vi "Enable Streaming.vi"(8 "error in (no error)":errorcluster, 11 "Node Ptr":T1 format="%.0x") -> (0 "error out":errorcluster)   [LabVIEW 2024, in "Nominal Client System Explorer.lvlib"]
uses:
  Nominal Client System Explorer.lvlib
  <vilib>/NI VeriStand/Custom Device API/Custom Device Item Ref.ctl
  <vilib>/NI VeriStand/Custom Device API/Custom Device API.lvlib
panel:
  in  "Specific Header":cluster{"Section Name":string}={"Section Name"="Specific Page Settings"}
  in  "General Header":cluster{"Section Name":string}={"Section Name"="General Page Settings"}
  in  "Description":string
  in  "Name":string
  # "Overview\nThe system provides a data channel that controls whether data is streamed to a file. This channel accepts float values but functions as a Boolean control.\n\nHow It Works\nChannel Value = 0: Streaming is disabled (False)\nChannel Value != 0: Streaming is enabled (True)\n\nUsage Methods\nManual Control\nPlace a Button on the User Interface screen and link it to:\n`Nominal IO VeriStand Client\\Enable Streaming`\nThis provides direct manual control over the streaming functionality.\n\nDynamic Control\nYou can also incorporate the channel in calculations to automatically control streaming based on other conditions or system states."
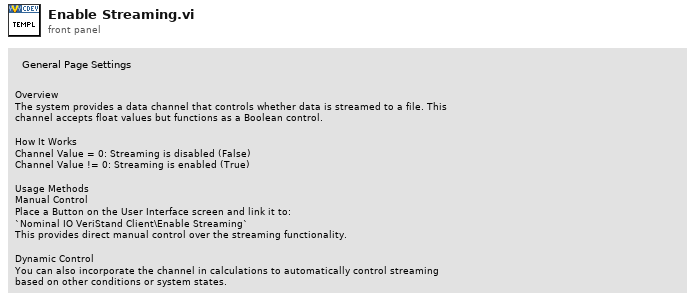
[diagram p1: front panel]
types:
  T1 = typedef "Custom Device API.lvlib/Custom Device Item Ref.ctl" = u64
  T2 = typedef "Custom Device API.lvlib/Custom Device Item Info.ctl" = cluster{"Name":string, "Is Channel":bool, "GUID":string, "Is Waveform":bool}
  T3 = typedef "Custom Device API.lvlib/Custom Device Commands.ctl" = enum16{"Default", "Item renamed", "Shutdown", "Dynamic button pressed"}
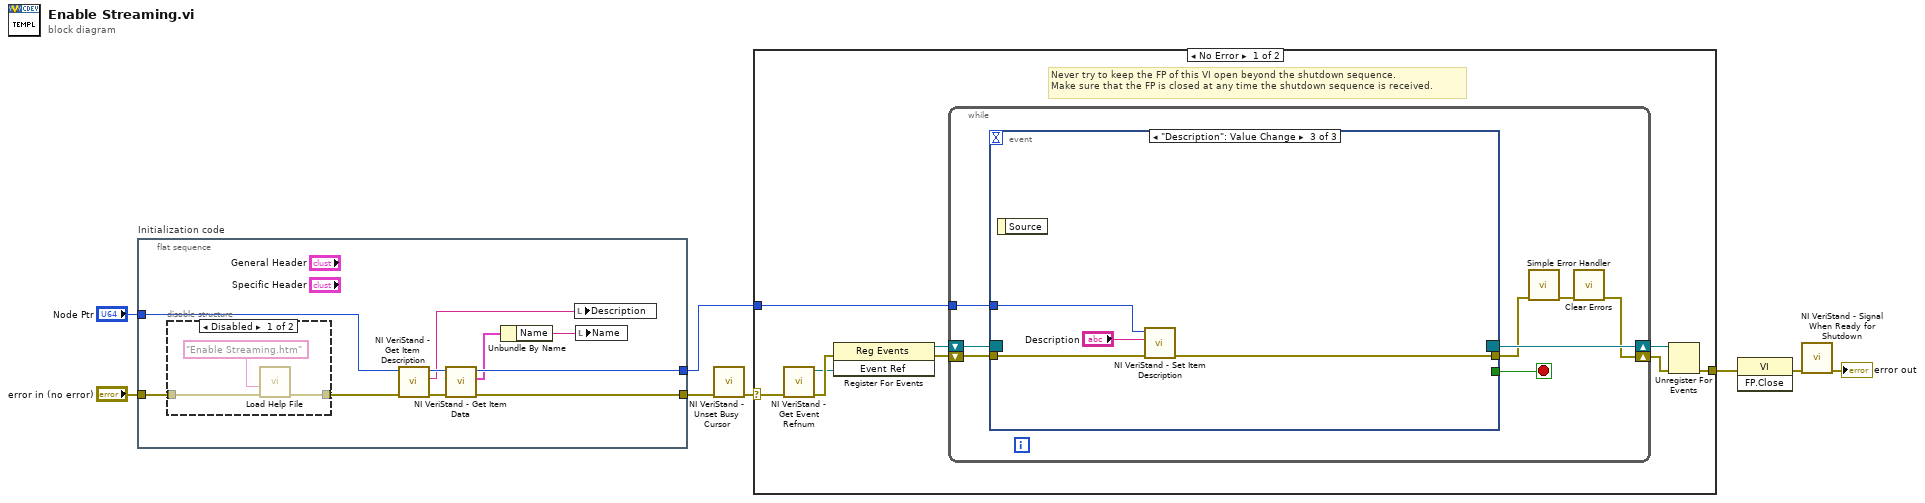
[diagram p0: block diagram]
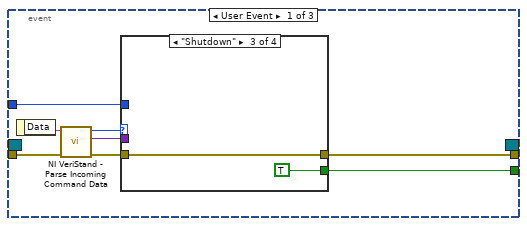
[diagram p2: hidden frame]
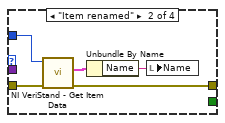
[diagram p4: hidden frame]
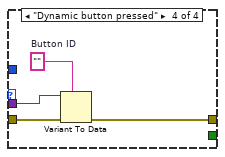
[diagram p5: hidden frame]
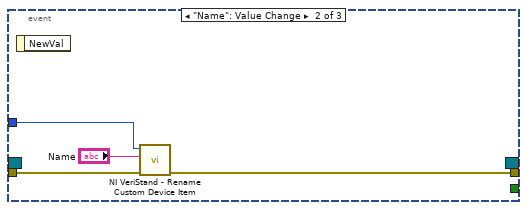
[diagram p6: hidden frame]
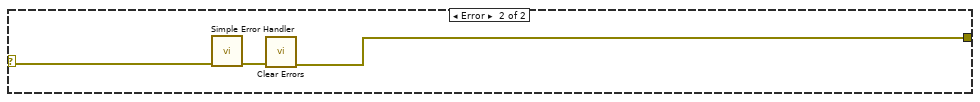
[diagram p7: hidden frame]
diagram:
  n1 = flat-sequence "Initialization code" {
    tunnel: "error in (no error)" -> [w10]
    tunnel: "Node Ptr" -> [w13]
    tunnel: [w14] -> w4
    tunnel: [w18] -> w1
    frame #0 {
      n2 = disable-structure shown="Disabled" {
        disable-tunnel: w10 -> [w21 w22]
        disable-tunnel: [w20 w22] -> w9
        frame Disabled {
          n3 = call "Load Help File.vi"("error in (no error)"=w21, "HTML File to Load"="Enable Streaming.htm" ("CD_CHM_Section")) -> ("error out"=w20:errorcluster)  [unwired: 9 in]
        }
        frame Enabled {
        }
      }
      n4 = call <vilib>:"NI VeriStand - Get Item Description.vi"("error in (no error)"=w9, "Item Ref in"=w13) -> ("error out"=w16:errorcluster, "Description"=w11:string, "Item Ref out"=w17:T1)  [unwired: 7 out]
      n5 = call <vilib>:"NI VeriStand - Get Item Data.vi"("error in (no error)"=w16, "Item Ref in"=w17) -> ("error out"=w14:errorcluster, "Item Info"=w15:T2, "Item Ref out"=w18:T1)  [unwired: 7 out]
      n6 = Unbundle By Name(w15) -> ("Name"=w12:string)
      n7 = local write "Description"(w11) -> ()
      n8 = local write "Name"(w12) -> ()
    }
  }
  n9 = call <vilib>:"NI VeriStand - Unset Busy Cursor.vi"("error in (no error)"=w4) -> ("error out"=w3:errorcluster)  [unwired: 10 out]
  n10 = case shown="No Error" w3 {
    selector: w3 -> [w23 w70]
    tunnel: [w28 w68] -> w8
    tunnel: w1 -> [w24 _]
    frame No Error {
      # "Never try to keep the FP of this VI open beyond the shutdown sequence.\nMake sure that the FP is closed at any time the shutdown sequence is received."
      n11 = call <vilib>:"NI VeriStand - Get Event Refnum.vi"("error in (no error)"=w23) -> ("error out"=w31:errorcluster, "Event Ref"=w27:refnum<user-event>)  [unwired: 9 out]
      n12 = register-events(error in=w31, w27) -> (reference out=w25:refnum<event-registration>, error out=w26:errorcluster)  [unwired: 1 in]
      n13 = while {
        tunnel: w24 -> [w35]
        shift-right: [w32] -> w29
        shift-left: w26 -> [w38]
        shift-right: [w39] -> w30
        shift-left: w25 -> [w37]
        stop <- w36 stop-if-true
        n14 = event shown="[2] \"Description\": Value Change" {
          selector: w37 -> [_ _ _]
          dyn-events: [_ _ _] -> w39
          timeout: _ -> [_ _ _]
          tunnel: w38 -> [w47 w63 w66]
          tunnel: [w43 _ _] -> w36
          tunnel: [w42 w62 w65] -> w34
          tunnel: w35 -> [w41 w61 w67]
          event User Event {
            n15 = event-data() -> ("Data"=w46:string)  [unwired: 1 out]
            n16 = call <vilib>:"NI VeriStand - Parse Incoming Command Data.vi"("error in (no error)"=w47, "Incoming data"=w46) -> ("error out"=w45:errorcluster, "Outgoing data"=w40:variant, "Action"=w44:T3)  [unwired: 7 out]
            n17 = case shown="\"Shutdown\"" w44 {
              tunnel: w45 -> [w48 w53 w54 w59]
              tunnel: [_ _ TRUE _] -> w43
              tunnel: [w48 w50 w54 w56] -> w42
              tunnel: w41 -> [_ w52 _ _]
              tunnel: w40 -> [_ _ _ w58]
              frame "Default", Default {
              }
              frame "Item renamed" {
                n18 = call <vilib>:"NI VeriStand - Get Item Data.vi"("error in (no error)"=w53, "Item Ref in"=w52) -> ("error out"=w50:errorcluster, "Item Info"=w51:T2)  [unwired: 8 out]
                n19 = Unbundle By Name(w51) -> ("Name"=w49:string)
                n20 = local write "Name"(w49) -> ()
              }
              frame "Shutdown" {
              }
              frame "Dynamic button pressed" {
                w57 = ""  # Button ID
                n21 = Variant To Data(error in=w59, type=w57, Variant=w58) -> (error out=w56:errorcluster)  [unwired: 1 out]
              }
            }
          }
          event "Name": Value Change {
            n22 = event-data() -> ()  [unwired: 2 out]
            n23 = call <vilib>:"NI VeriStand - Rename Custom Device Item.vi"("error in (no error)"=w63, "New Name"="Name", "Item Ref in"=w61) -> ("error out"=w62:errorcluster)  [unwired: 1 in, 7 out]
          }
          event "Description": Value Change {
            n24 = event-data() -> ()  [unwired: 2 out]
            n25 = call <vilib>:"NI VeriStand - Set Item Description.vi"("error in (no error)"=w66, "Description"="Description", "Item Ref in"=w67) -> ("error out"=w65:errorcluster)  [unwired: 8 out]
          }
        }
        n26 = call <vilib>:"Simple Error Handler.vi"("error in (no error)"=w34) -> ("error out"=w33:errorcluster)  [unwired: 1 in, 7 out]
        n27 = call <vilib>:"Clear Errors.vi"("error in (no error)"=w33) -> ("error out"=w32:errorcluster)  [unwired: 1 in, 5 out]
      }
      n28 = Unregister For Events(event registration refnum=w30, error in=w29) -> (error out=w28:errorcluster)
    }
    frame Error {
      n29 = call <vilib>:"Simple Error Handler.vi"("error in (no error)"=w70) -> ("error out"=w69:errorcluster)  [unwired: 1 in, 7 out]
      n30 = call <vilib>:"Clear Errors.vi"("error in (no error)"=w69) -> ("error out"=w68:errorcluster)  [unwired: 1 in, 5 out]
    }
  }
  n31 = invoke class="VI" method="FP.Close"(error in=w8) -> (error out=w7:errorcluster)  [unwired: 2 in, 2 out]
  n32 = call <vilib>:"NI VeriStand - Signal When Ready for Shutdown.vi"("error in (no error)"=w7) -> ("error out"=→"error out":errorcluster)  [unwired: 10 out]
